vi "Mapping Arrays Different Length.vi"   [LabVIEW 2016, in "System Mapping Tool.lvlib"]
uses:
  System Mapping Tool.lvlib
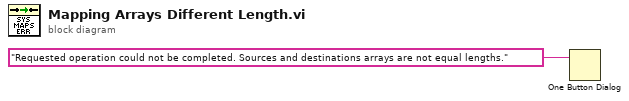
[diagram p0: block diagram]
diagram:
  n1 = One Button Dialog(message="Requested operation could not be completed. Sources and destinations arrays are not equal lengths.") -> ()  [unwired: 1 in, 1 out]
